vi "StringToJSON.vi"(11 "input text":string) -> (3 "JSON string":string)   [LabVIEW 2019]
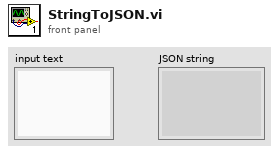
[diagram p1: front panel]
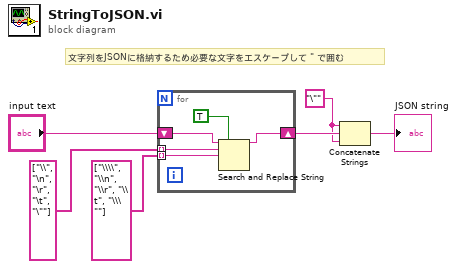
[diagram p0: block diagram]
diagram:
  w1 = "\"" ("string")
  # "文字列をJSONに格納するため必要な文字をエスケープして \" で囲む"
  n1 = for {
    shift-right: [w11] -> w3
    shift-left: "input text" -> [w10]
    tunnel: string[] ["\\", "\n", "\r", "\t", "\""] -> [w9] mode=indexing
    tunnel: string[] ["\\\\", "\\n", "\\r", "\\t", "\\\""] -> [w8] mode=indexing
    n2 = Search and Replace String(replace all?=TRUE ("replace all? (F)"), input string=w10, search string=w9, replace string=w8) -> (result string=w11:string)  [unwired: 4 in, 3 out]
  }
  n3 = Concatenate Strings(w1, w3, w1) -> (→"JSON string":string)
